vi "Op-Graphics-Overlay.vi"(8 "error in (no error)":errorcluster, 9 "size to present scale":bool, 10 "overlay plane (off:0)":u8(ring) items=["off", "memory 1", "memory 2", "memory 3", "memory 4"], 11 "VISA session":refnum<visa-resource-name>) -> (0 "error out":errorcluster, 3 "VISA resource name out":refnum<visa-resource-name>)   [LabVIEW 2016, in "Agilent 415X Series.lvlib"]
doc: "This VI controls the use of overlay planes. Up to four traces can be stored in the internal memory. After recalling a trace, providing it exists, the user may force the scale of the present measurement data to that of the overlay plane. Overlay plane information is show automatically."
uses:
  Agilent 415X Series.lvlib
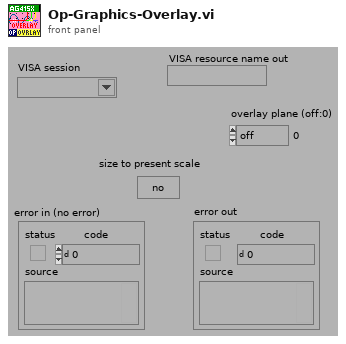
[diagram p1: front panel]
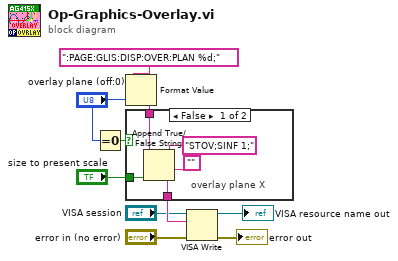
[diagram p0: block diagram]
diagram:
  n1 = Equal To 0?(x="overlay plane (off:0)") -> (x = 0?=w7:bool)
  n2 = Format Value(format string=":PAGE:GLIS:DISP:OVER:PLAN %d;", value (0)="overlay plane (off:0)") -> (output string=w10:string)  [unwired: 1 in]
  n3 = case shown="False" w7 {
    tunnel: w10 -> [w14 w16]
    tunnel: "size to present scale" -> [w15 _]
    tunnel: [w12 w16] -> w5
    frame False {
      # "overlay plane X"
      n4 = Append True/False String(1:w15, 2:"", 3:"STOV;SINF 1;", 4:w14) -> (0:w12:string)
    }
    frame True {
      # "overlay plane off"
    }
  }
  n5 = VISA Write(VISA resource name="VISA session", write buffer=w5, error in (no error)="error in (no error)") -> (VISA resource name out=→"VISA resource name out":refnum<visa-resource-name>, error out=→"error out":errorcluster)  [unwired: 1 out]
